vi "clearAllHandshakes.vi"   [LabVIEW 2014]
uses:
  <vilib>/Platform/TimedLoop/XDataNode/timing_clust.ctl
  <vilib>/Platform/TimedLoop/XDataNode/nitl_modes.ctl
  <vilib>/Platform/TimedLoop/XDataNode/wakeup.ctl
  <vilib>/rvi/Emulation/niFpgaSctlEmulationGetInTimedLoop.vi
  <vilib>/rvi/Emulation/niFpgaEmulationReportErrorSimple.vi
  <vilib>/rvi/Emulation/niFpgaGetClockAttributes.vi
  <vilib>/rvi/Emulation/niFpgaCriticalErrorInLSC.vi
  <vilib>/rvi/Emulation/niFpgaEmulationIsFPGAContextNoSignature.vi
  <vilib>/rvi/DataTransferAndStorage/Container/Common/niFpgaContainerGetUniqueNameForEmu.vi
  <vilib>/rvi/eio/common/nirviEmuReportErrorAndStop.vi
  <vilib>/rvi/Emulation/niFpgaProcessEmulError.vi
  <vilib>/Platform/TimedLoop/XDataNode/XDataNode.xnode
  <vilib>/rvi/DataTransferAndStorage/Container/XNode/niFpgaContainer.xnode
  <vilib>/rvi/DataTransferAndStorage/Handshake/Emulation/niFpgaHandshakeEmulation.vi
  <vilib>/Platform/TimedLoop/XDataNode/XDNodeRunTimeDep.lvlib
types:
  T1 = typedef "XDNodeRunTimeDep.lvlib/timing_clust.ctl" = cluster{"Expected End [f-1]":u64, "Actual End [f-1]":u64, "Finished Late? [f-1]":bool, "Expected End [i-1]":u64, "Actual End [i-1]":u64, "Finished Late? [i-1]":bool, "Expected Start [i]":u64, "Actual Start [i]":u64, "Expected Start [f]":u64, "Actual Start [f]":u64, "Source Name":string, "Structure Name":string, "Period":i64, "Deadline":i64, "Offset":i64, "Start":i64, "Priority":i32, "Timeout":i32, "Mode":T2, "Wakeup Reason":T3, "Error":errorcluster, "Source Type":string, "Secondary Source Type":string, "Global End Time":u64, "Global Start Time":u64, "Frame Duration":u64, "Iteration Duration":u64, "Assigned CPU":i32, "I/O Scan Engine Mode":u32}
  T2 = typedef "XDNodeRunTimeDep.lvlib/nitl_modes.ctl" = enum32{"No Change", "Process missed periods, maintain original phase", "Discard missed periods, maintain original phase", "Process missed periods, ignore original phase", "Discard missed periods, ignore original phase"}
  T3 = typedef "XDNodeRunTimeDep.lvlib/wakeup.ctl" = enum32{"Normal", "Aborted", "Asynchronous wakeup", "Timing source error", "Timed loop error", "Timeout"}
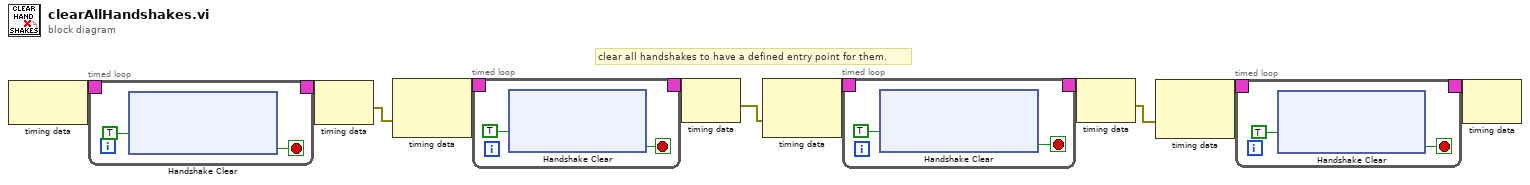
[diagram p0: block diagram]
diagram:
  # "clear all handshakes to have a defined entry point for them."
  n1 = node-c288() -> (w11:T1)  [unwired: 1 in]
  n2 = timed-loop {
    timing: w11 -> [_]
    timing-out: [_] -> w10
    stop <- w12 stop-if-true
    n3 = xnode ("Handshake Clear")("Start"=TRUE) -> ("Done"=w12:bool)  [unwired: 1 in, 1 out]
  }
  n4 = node-c288(w10) -> (w7:errorcluster)
  n5 = node-c288(w7) -> (w9:T1)  [unwired: 1 in]
  n6 = timed-loop {
    timing: w9 -> [_]
    timing-out: [_] -> w8
    stop <- w17 stop-if-true
    n7 = xnode ("Handshake Clear")("Start"=TRUE) -> ("Done"=w17:bool)  [unwired: 1 in, 1 out]
  }
  n8 = node-c288(w8) -> (w4:errorcluster)
  n9 = node-c288(w4) -> (w6:T1)  [unwired: 1 in]
  n10 = timed-loop {
    timing: w6 -> [_]
    timing-out: [_] -> w5
    stop <- w21 stop-if-true
    n11 = xnode ("Handshake Clear")("Start"=TRUE) -> ("Done"=w21:bool)  [unwired: 1 in, 1 out]
  }
  n12 = node-c288(w5) -> (w1:errorcluster)
  n13 = node-c288(w1) -> (w3:T1)  [unwired: 1 in]
  n14 = timed-loop {
    timing: w3 -> [_]
    timing-out: [_] -> w2
    stop <- w25 stop-if-true
    n15 = xnode ("Handshake Clear")("Start"=TRUE) -> ("Done"=w25:bool)  [unwired: 1 in, 1 out]
  }
  n16 = node-c288(w2) -> ()  [unwired: 1 out]
